vi "Add Plugin with Children.vi"(8 "error in (no error)":errorcluster, 9 "Plugin":refnum<class "Plugin.lvclass">, 10 "parent tag":string, 11 "Application Data In":T1) -> (0 "error out":errorcluster, 2 "average bandwidth":dbl, 3 "Application Data Out":T1)   [LabVIEW 2017, in "DSF Core.lvlib"]
uses:
  DSF Core.lvlib
  Main VI/Application Data.ctl
  <vilib>/NI/Memory Manager/Classes/Pointer/Pointer.lvclass
  Classes/Framework/Framework.lvclass
  Buffer Reader/Buffer Data.ctl
  Classes/Buffer/Buffer.lvclass
  C:/Program Files (x86)/National Instruments/LabVIEW 2017/vi.lib/NI/Memory Manager/Classes/Pointer/Pointer.lvclass
  Classes/Transfer Group Status/Status.lvclass
  Typedefs/DSF Engine Framework Configuration.ctl
  Typedefs/DSF Engine Plugin Configuration.ctl
  Typedefs/DSF Timing Info.ctl
  Typedefs/DSF Engine Plugin Thread Configuration.ctl
  Typedefs/DSF Settings Info.ctl
  Typedefs/DSF Engine Transfer Group Configuration.ctl
  Typedefs/DSF Direction.ctl
  Typedefs/DSF Engine Transfer Configuration.ctl
  Typedefs/DSF Byte Order.ctl
  Typedefs/DSF Engine Channel Configuration.ctl
  Typedefs/DSF Data Type.ctl
  Typedefs/DSF Timeout Behavior.ctl
  Classes/Plugin/Plugin.lvclass
  Classes/Plugin/Plugin.lvclass/Plugin.ctl
  Classes/Buffers/Buffers.lvclass/Buffers.ctl
  Classes/Timing/Timing.lvclass/Timing.ctl
  ID to Tree Items/Tree Item Type.ctl
  Classes/Transfer Group/Transfer Group.lvclass/Transfer Group.ctl
  <vilib>/NI/Memory Manager/Classes/Pointer/Pointer.lvclass/Pointer.ctl
  Classes/Transfer/Transfer.lvclass/Transfer.ctl
  Add Transfer.vi
  Classes/Transfer Group/Get Transfers.vi
  Classes/Transfer Group/Get Inline.vi
  Buffer Reader/Average Cycle Bandwidth.vi
  Add Buffers.vi
  Classes/Buffer/Get Buffer Size.vi
  Classes/Buffers/Get Async Buffer.vi
  Classes/Buffers/Get Inline Buffer.vi
  <vilib>/NI/Memory Manager/Classes/Pointer/Get Size.vi
  Classes/Timing/Timing.lvclass
  Classes/Buffers/Buffers.lvclass
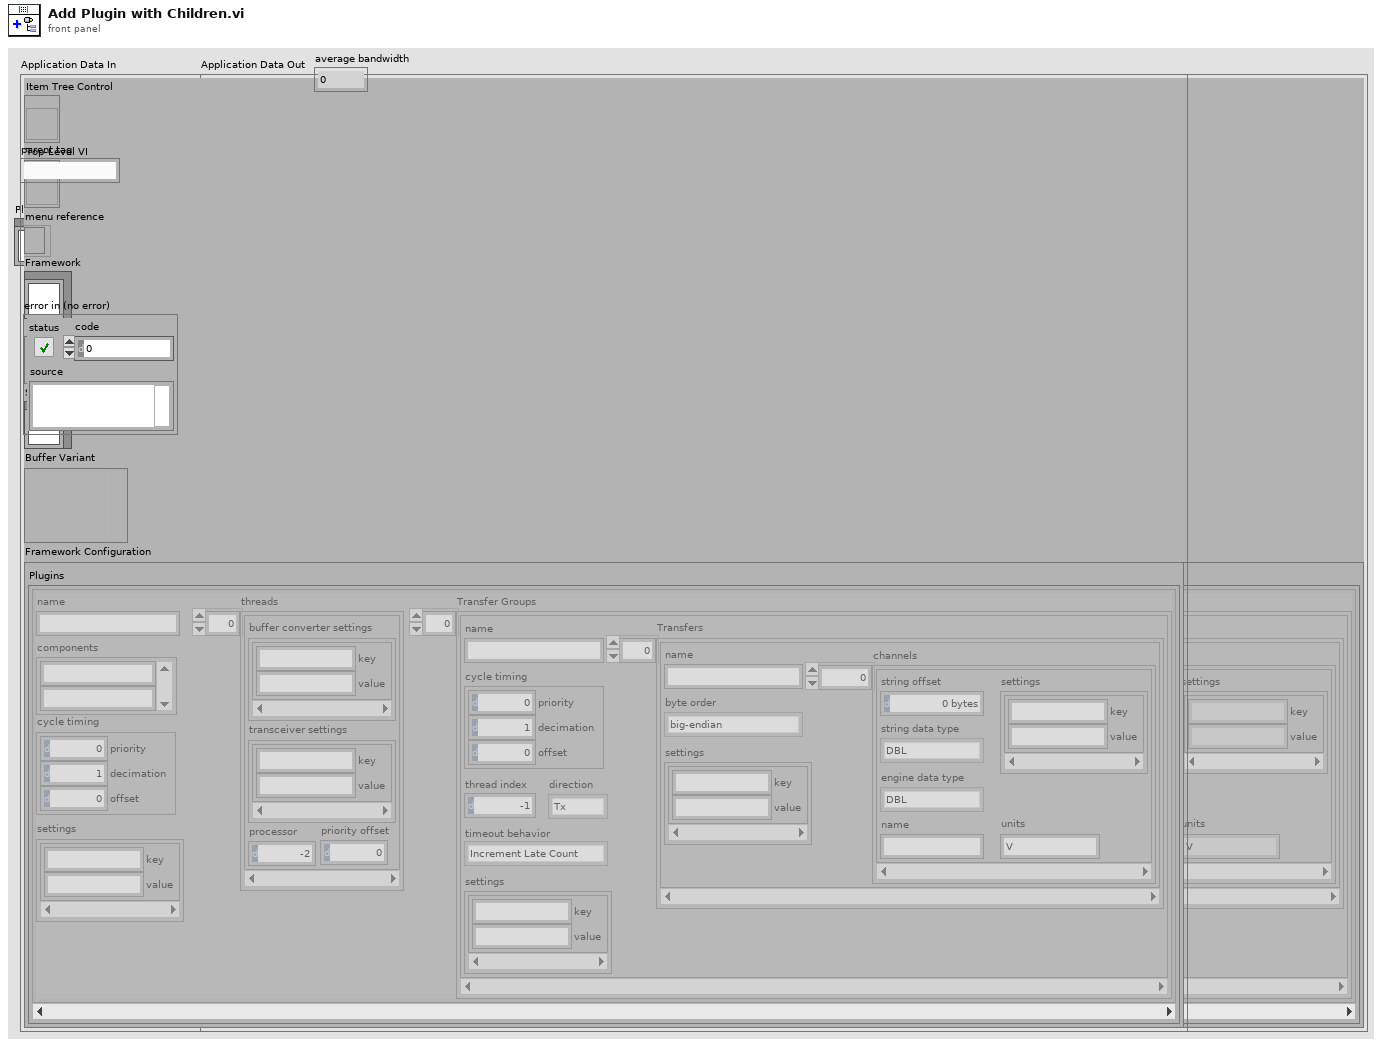
[diagram p1: front panel]
types:
  T1 = typedef "DSF Core.lvlib/Application Data.ctl" = cluster{"Item Tree Control":refnum<vi>, "Top-Level VI":refnum<vi>, "menu reference":refnum<k9>, "Framework":refnum<class "Framework.lvclass">, "buffer queue":refnum<queue>, "Stop Pointer":refnum<class "Pointer.lvclass">, "Buffer Variant":variant, "Framework Configuration":T2}
  T2 = typedef "DSF Core.lvlib/DSF Engine Framework Configuration.ctl" = cluster{"Plugins":T3[]}
  T3 = typedef "DSF Core.lvlib/DSF Engine Plugin Configuration.ctl" = cluster{"name":string, "components":string[], "cycle timing":T4, "threads":T5[], "Transfer Groups":T7[], "settings":T6}
  T4 = typedef "DSF Core.lvlib/DSF Timing Info.ctl" = cluster{"priority":u64, "decimation":u64, "offset":u64}
  T5 = typedef "DSF Core.lvlib/DSF Engine Plugin Thread Configuration.ctl" = cluster{"buffer converter settings":T6, "transceiver settings":T6, "processor":i32, "priority offset":i16}
  T6 = typedef "DSF Core.lvlib/DSF Settings Info.ctl" = cluster{"key":string, "value":string}[]
  T7 = typedef "DSF Core.lvlib/DSF Engine Transfer Group Configuration.ctl" = cluster{"name":string, "direction":T8, "cycle timing":T4, "thread index":i32, "settings":T6, "Transfers":T9[], "timeout behavior":T13}
  T8 = typedef "DSF Core.lvlib/DSF Direction.ctl" = enum8{"Tx", "Rx"}
  T9 = typedef "DSF Core.lvlib/DSF Engine Transfer Configuration.ctl" = cluster{"name":string, "byte order":T10, "settings":T6, "channels":T11[]}
  T10 = typedef "DSF Core.lvlib/DSF Byte Order.ctl" = enum8{"big-endian", "little-endian"}
  T11 = typedef "DSF Core.lvlib/DSF Engine Channel Configuration.ctl" = cluster{"string offset":u64, "string data type":T12, "engine data type":T12, "name":string, "settings":T6, "units":string}
  T12 = typedef "DSF Core.lvlib/DSF Data Type.ctl" = enum8{"Bool", "SGL", "DBL", "I8", "I16", "I32", "I64", "U8", "U16", "U32", "U64"}
  T13 = typedef "DSF Core.lvlib/DSF Timeout Behavior.ctl" = enum8{"Increment Late Count", "Throw Error"}
  T14 = typedef "DSF Core.lvlib/Buffer Data.ctl" = cluster{"Buffer":refnum<class "Buffer.lvclass">, "Status":refnum<class "Status.lvclass">, "decimation":u64, "avg bandwidth":dbl}
  T15 = typedef "DSF Core.lvlib/Tree Item Type.ctl" = enum16{"Framework", "Plugin Group", "Plugin", "Group", "Transfer", "Buffer", "Channel"}
  T16 = typedef "DSF Core.lvlib/Tree Item.ctl" = cluster{"Left Cell String":string, "Child Text":string[], "Child Tag":string, "Glyph Index":i32}
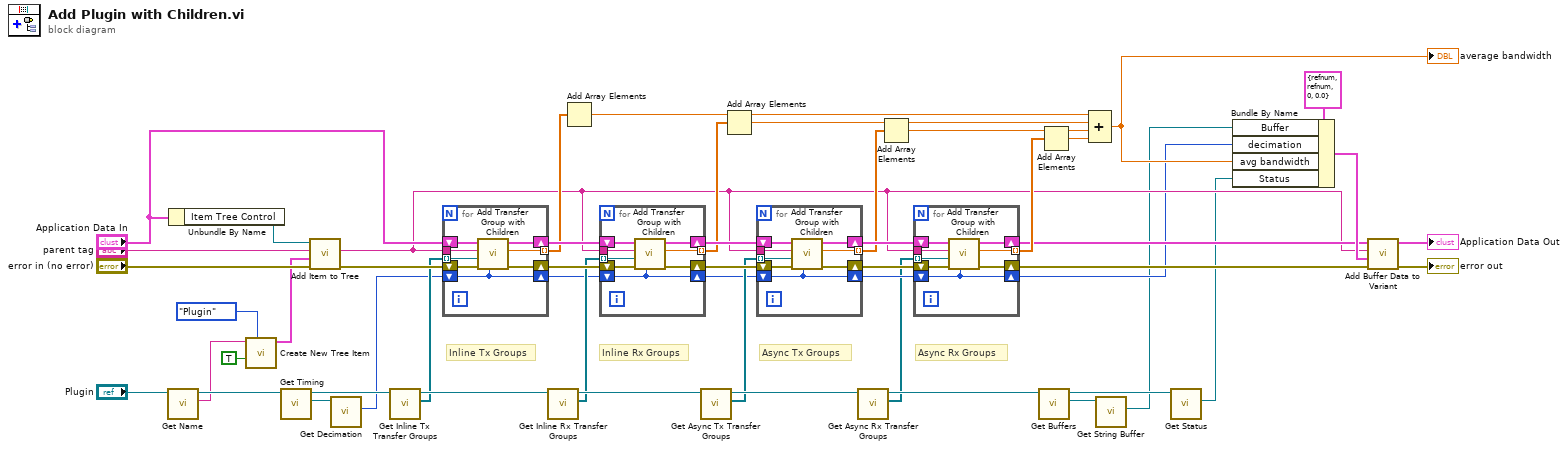
[diagram p0: block diagram]
diagram:
  # "Async Rx Groups"
  # "Async Tx Groups"
  # "Inline Rx Groups"
  # "Inline Tx Groups"
  n1 = call "Get Name.vi"("Plugin in"="Plugin") -> ("name"=w24:string, "Plugin out"=w25:refnum<class "Plugin.lvclass">)  [unwired: 9 in]
  n2 = Unbundle By Name("Application Data In") -> ("Item Tree Control"=w36:refnum<vi>)
  n3 = call "Create New Tree Item.vi"("Item Type"=Tree_Item_Type."Plugin", "found?"=TRUE, "Left Cell String"=w24) -> ("Item"=w45:T16)  [unwired: 7 in, 1 out]
  n4 = call "Get Timing.vi"("Plugin in"=w25) -> ("Timing"=w22:refnum<class "Timing.lvclass">, "Plugin out"=w23:refnum<class "Plugin.lvclass">)  [unwired: 9 in]
  n5 = call "Add Item to Tree.vi"("error in (no error)"="error in (no error)", "Item"=w45, "parent tag"="parent tag", "TreeControl in"=w36) -> ("error out"=w27:errorcluster, "new item tag"=w7:string)  [unwired: 5 in, 1 out]
  n6 = call "Get Decimation.vi"("Timing in"=w22) -> ("Decimation"=w4:u64)  [unwired: 9 in, 1 out]
  n7 = call "Get Inline Tx Transfer Groups.vi"("Plugin in"=w23) -> ("Inline Tx Transfer Groups"=w26:refnum<class "Transfer Group.lvclass">[], "Plugin out"=w48:refnum<class "Plugin.lvclass">)  [unwired: 9 in]
  n8 = for {
    tunnel: w7 -> [w55]
    tunnel: w26 -> [w56] mode=indexing
    shift-right: [w57] -> w44
    shift-left: "Application Data In" -> [w60]
    shift-right: [w58] -> w43
    shift-left: w27 -> [w59]
    shift-right: [w54] -> w31
    shift-left: w4 -> [w54]
    tunnel: [w53] -> w14 mode=indexing
    # "Inline Tx Groups"
    n9 = call "Add Transfer Group with Children.vi"("Plugin Decimation (1)"=w54, "error in (no error)"=w59, "Transfer Group"=w56, "parent tag"=w55, "Application Data In"=w60) -> ("error out"=w58:errorcluster, "average bandwidth"=w53:dbl, "Application Data In"=w57:T1)  [unwired: 4 in]
  }
  n10 = call "Get Inline Rx Transfer Groups.vi"("Plugin in"=w48) -> ("Inline Rx Transfer Groups"=w38:refnum<class "Transfer Group.lvclass">[], "Plugin out"=w47:refnum<class "Plugin.lvclass">)  [unwired: 9 in]
  n11 = Add Array Elements(numeric array=w14) -> (sum=w18:dbl)
  n12 = for {
    tunnel: w7 -> [w63]
    tunnel: w38 -> [w64] mode=indexing
    shift-right: [w65] -> w42
    shift-left: w44 -> [w68]
    shift-right: [w66] -> w41
    shift-left: w43 -> [w67]
    shift-right: [w62] -> w30
    shift-left: w31 -> [w62]
    tunnel: [w61] -> w21 mode=indexing
    # "Inline Rx Groups"
    n13 = call "Add Transfer Group with Children.vi"("Plugin Decimation (1)"=w62, "error in (no error)"=w67, "Transfer Group"=w64, "parent tag"=w63, "Application Data In"=w68) -> ("error out"=w66:errorcluster, "average bandwidth"=w61:dbl, "Application Data In"=w65:T1)  [unwired: 4 in]
  }
  n14 = call "Get Async Tx Transfer Groups.vi"("Plugin in"=w47) -> ("Async Tx Transfer Groups"=w37:refnum<class "Transfer Group.lvclass">[], "Plugin out"=w46:refnum<class "Plugin.lvclass">)  [unwired: 9 in]
  n15 = Add Array Elements(numeric array=w21) -> (sum=w17:dbl)
  n16 = for {
    tunnel: w7 -> [w71]
    tunnel: w37 -> [w72] mode=indexing
    shift-right: [w73] -> w40
    shift-left: w42 -> [w76]
    shift-right: [w74] -> w39
    shift-left: w41 -> [w75]
    shift-right: [w70] -> w29
    shift-left: w30 -> [w70]
    tunnel: [w69] -> w20 mode=indexing
    # "Async Tx Groups"
    n17 = call "Add Transfer Group with Children.vi"("Plugin Decimation (1)"=w70, "error in (no error)"=w75, "Transfer Group"=w72, "parent tag"=w71, "Application Data In"=w76) -> ("error out"=w74:errorcluster, "average bandwidth"=w69:dbl, "Application Data In"=w73:T1)  [unwired: 4 in]
  }
  n18 = call "Get Async Rx Transfer Groups.vi"("Plugin in"=w46) -> ("Async Rx Transfer Groups"=w6:refnum<class "Transfer Group.lvclass">[], "Plugin out"=w13:refnum<class "Plugin.lvclass">)  [unwired: 9 in]
  n19 = Add Array Elements(numeric array=w20) -> (sum=w16:dbl)
  n20 = for {
    tunnel: w7 -> [w79]
    tunnel: w6 -> [w80] mode=indexing
    shift-right: [w81] -> w11
    shift-left: w40 -> [w84]
    shift-right: [w82] -> w9
    shift-left: w39 -> [w83]
    shift-right: [w78] -> w5
    shift-left: w29 -> [w78]
    tunnel: [w77] -> w19 mode=indexing
    # "Async Rx Groups"
    n21 = call "Add Transfer Group with Children.vi"("Plugin Decimation (1)"=w78, "error in (no error)"=w83, "Transfer Group"=w80, "parent tag"=w79, "Application Data In"=w84) -> ("error out"=w82:errorcluster, "average bandwidth"=w77:dbl, "Application Data In"=w81:T1)  [unwired: 4 in]
  }
  n22 = call "Get Buffers.vi"("Plugin in"=w13) -> ("Buffers"=w32:refnum<class "Buffers.lvclass">, "Plugin out"=w3:refnum<class "Plugin.lvclass">)  [unwired: 9 in]
  n23 = Add Array Elements(numeric array=w19) -> (sum=w15:dbl)
  n24 = Compound Arithmetic op=ADD(w18, w17, w16, w15) -> (w12:dbl)
  "average bandwidth" <- w12
  n25 = call "Get String Buffer.vi"("Buffers in"=w32) -> ("String Buffer"=w1:refnum<class "Buffer.lvclass">)  [unwired: 9 in, 1 out]
  n26 = call "Get Status.vi"("Plugin in"=w3) -> ("status pointer"=w2:refnum<class "Status.lvclass">)  [unwired: 9 in, 1 out]
  n27 = Bundle By Name(cluster=T14 {"Buffer"=refnum, "Status"=refnum, "decimation"=0, "avg bandwidth"=0.0} ("Buffer data"), "Buffer"=w1, "decimation"=w5, "avg bandwidth"=w12, "Status"=w2) -> (w33:T14)
  n28 = call "Add Buffer Data to Variant.vi"("error in (no error)"=w9, "Buffer data"=w33, "tag"=w7, "Application Data In in"=w11) -> ("error out"=→"error out":errorcluster, "Application Data In out"=→"Application Data Out":T1)  [unwired: 6 in]
